vi "add new empty sequence.vi"(8 "error in (no error)":errorcluster, 10 "sequence name":string, 11 "Simple Sequencer TBM configuration in":refnum<class "Simple Sequencer TBM configuration.lvclass">) -> (0 "error out":errorcluster, 3 "Simple Sequencer TBM configuration out":refnum<class "Simple Sequencer TBM configuration.lvclass">)   [LabVIEW 2015, in "Simple Sequencer TBM configuration.lvclass"]
doc: "Creates a new empty sequence with the specifed sequence name."
uses:
  Simple Sequencer TBM configuration.lvclass
  Simple Sequencer TBM configuration.lvclass/Simple Sequencer TBM configuration.ctl
  sequence definition.ctl
  sequencer parent classes/action configuration parent/action configuration.lvclass
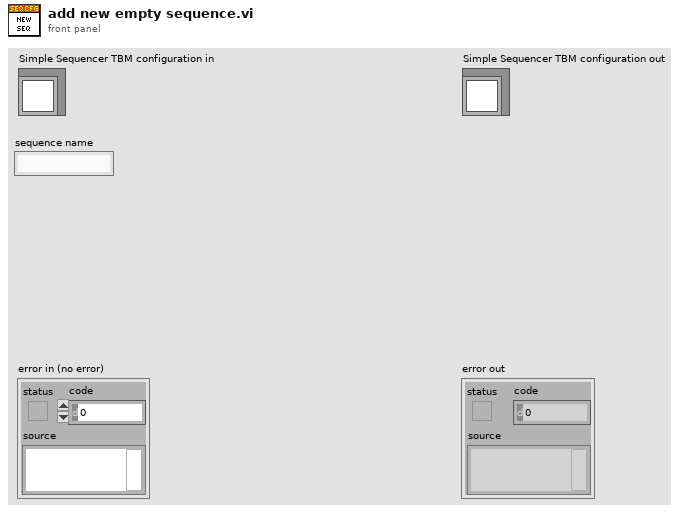
[diagram p1: front panel]
types:
  T1 = typedef "Simple Sequencer TBM configuration.lvclass/sequence definition.ctl" = cluster{"sequence name":string, "action configs":refnum<class "action configuration.lvclass">[]}
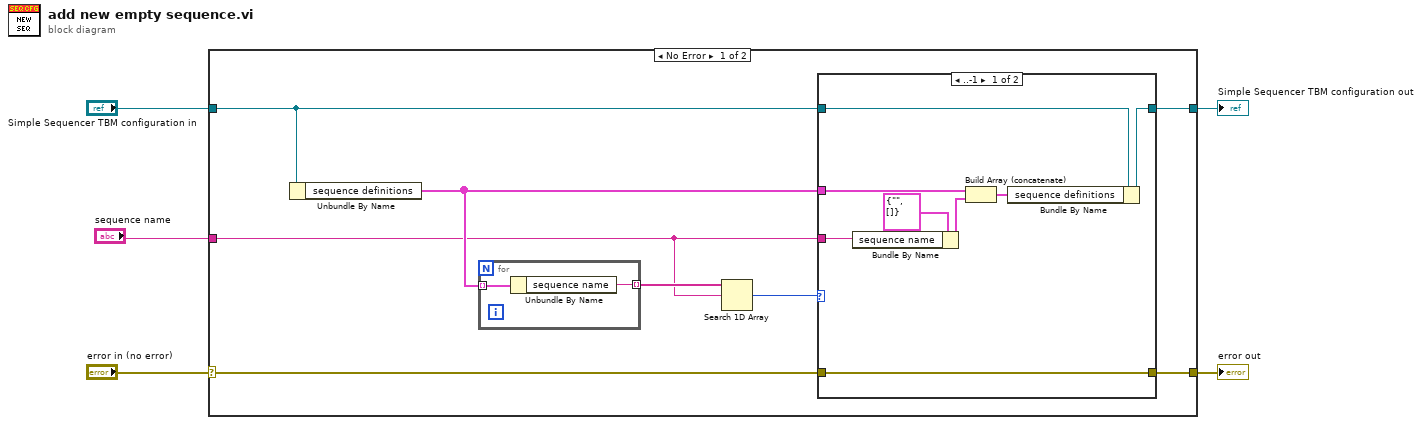
[diagram p0: block diagram]
diagram:
  n1 = case shown="No Error" "error in (no error)" {
    selector: "error in (no error)" -> [w7 w27]
    tunnel: [w6 w27] -> w4
    tunnel: [w12 w26] -> w2
    tunnel: "Simple Sequencer TBM configuration in" -> [w13 w26]
    tunnel: "sequence name" -> [w9 _]
    frame No Error {
      n2 = Unbundle By Name(w13) -> ("sequence definitions"=w11:T1[])
      n3 = for {
        tunnel: w11 -> [w25] mode=indexing
        tunnel: [w24] -> w10 mode=indexing
        n4 = Unbundle By Name(w25) -> ("sequence name"=w24:string)
      }
      n5 = Search 1D Array(1D array=w10, element=w9) -> (index of element=w8:i32)  [unwired: 1 in]
      n6 = case shown="..-1" w8 {
        tunnel: w13 -> [w19 w23]
        tunnel: [w17 w23] -> w12
        tunnel: w11 -> [w16 _]
        tunnel: w9 -> [w15 _]
        tunnel: w7 -> [w14 w22]
        tunnel: [w14 w22] -> w6
        frame ..-1 {
          n7 = Bundle By Name(cluster=T1 {"sequence name"="", "action configs"=[]} ("sequence definitions"), "sequence name"=w15) -> (w20:T1)
          n8 = Build Array (concatenate)(w16, w20) -> (w18:T1[])
          n9 = Bundle By Name(cluster=w19, "sequence definitions"=w18) -> (w17:refnum<class "Simple Sequencer TBM configuration.lvclass">)
        }
        frame 0.. {
          # "#todo throw error that a seq with this name already exists"
        }
      }
    }
    frame Error {
    }
  }
  "error out" <- w4
  "Simple Sequencer TBM configuration out" <- w2
